vi "rateCorrector.vi"(8 "threshold":dbl(slide) scale=0.0..25.0, 9 "intergration":dbl, 10 "count":dbl, 11 "HR":dbl) -> (0 "skipped":bool, 1 "error count":dbl, 2 "actual threshold":dbl, 3 "HR":dbl, 4 "Raw corr":dbl)   [LabVIEW 2010]
uses:
  <vilib>/ptbypt/NI_PtbyPt.lvlib
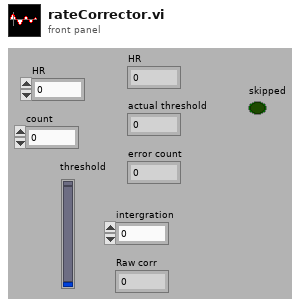
[diagram p1: front panel]
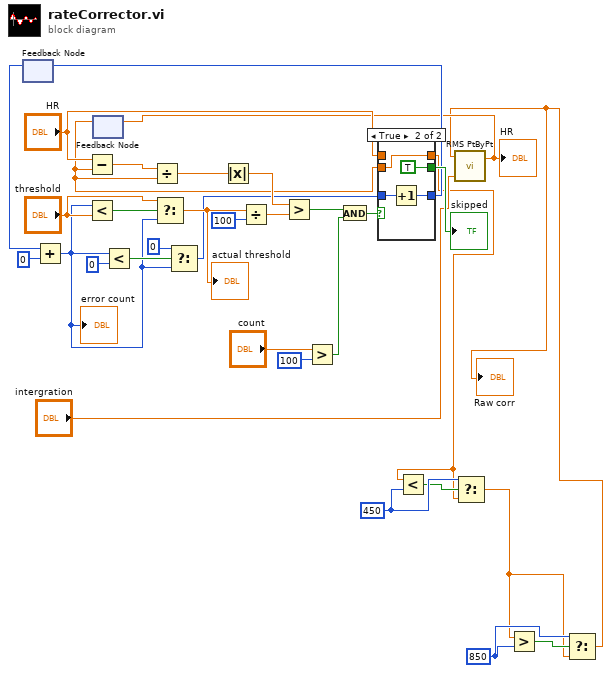
[diagram p0: block diagram]
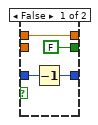
[diagram p2: hidden frame]
diagram:
  w3 = 850
  w7 = 450
  n1 = feedback #1() -> (w10:i32)  [unwired: 1 in]
  n2 = Add(x=w10, y=0) -> (x+y=w14:i32)
  "error count" <- w14
  n3 = Less?(x=w14, y="threshold") -> (x < y?=w21:bool)
  n4 = feedback #2() -> (w12:dbl)  [unwired: 1 in]
  n5 = Subtract(x="HR", y=w12) -> (x-y=w30:dbl)
  n6 = Less?(x=w14, y=0) -> (x < y?=w15:bool)
  n7 = Divide(x=w30, y=w12) -> (x/y=w29:dbl)
  n8 = Select(t="threshold", s=w21, f=w14) -> (s? t:f=w18:dbl)
  "actual threshold" <- w18
  n9 = Select(t=0, s=w15, f=w14) -> (s? t:f=w13:i32)
  n10 = Absolute Value(x=w29) -> (abs(x)=w28:dbl)
  n11 = Divide(x=w18, y=100) -> (x/y=w24:dbl)
  n12 = Greater?(x=w28, y=w24) -> (0:w27:bool)
  n13 = Greater?(x="count", y=100) -> (0:w19:bool)
  n14 = And(x=w27, y=w19) -> (x .and. y?=w26:bool)
  n15 = case shown="True" w26 {
    tunnel: [w37 w38] -> w5
    tunnel: "HR" -> [w37 _]
    tunnel: [FALSE TRUE] -> w25
    tunnel: [w35 w40] -> w11
    tunnel: w13 -> [w34 w39]
    tunnel: w12 -> [_ w38]
    frame False {
      n16 = Decrement(x=w34) -> (x-1=w35:i32)
    }
    frame True {
      n17 = Increment(x=w39) -> (x+1=w40:i32)
    }
  }
  "skipped" <- w25
  n18 = feedback-in #1(w11) -> ()
  n19 = Less?(x=w5, y=w7) -> (x < y?=w6:bool)
  n20 = Select(t=w7, s=w6, f=w5) -> (s? t:f=w2:dbl)
  n21 = Greater?(x=w2, y=w3) -> (0:w4:bool)
  n22 = Select(t=w3, s=w4, f=w2) -> (s? t:f=w1:dbl)
  "Raw corr" <- w1
  n23 = call <vilib>:"RMS PtByPt.vi"("sample length"="intergration", "x"=w1) -> ("rms value"=w9:dbl)  [unwired: 2 in, 1 out]
  "HR" <- w9
  n24 = feedback-in #2(w9) -> ()
